vi "Hyperbolic Sine Integral.vi"(3 "x":dbl format="%.2f") -> (1 "Shi(x)":dbl format="%.2f")   [LabVIEW 2020, in "NI_Gmath.lvlib"]
doc: "Computes the hyperbolic sine integral function."
uses:
  NI_Gmath.lvlib
  <resource>/lvanlys.dll
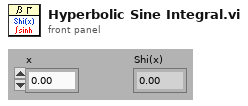
[diagram p1: front panel]
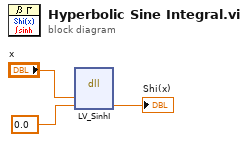
[diagram p0: block diagram]
diagram:
  n1 = dll-call lib="C:/Program Files (x86)/National Instruments/LabVIEW 2020/resource/lvanlys.*" fn="LV_SinhI"("x"="x", "SinhI(x)"=0.0 ("cosI")) -> ("SinhI(x)"=→"Shi(x)":dbl)  [unwired: 5 in, 2 out]
